vi "Rotation stage shgv2.vi"() -> ()   [LabVIEW 2020]
doc: "Shows how to move a motor to an absolute position."
uses:
  <vilib>/Utility/error.llb/DialogType.ctl
  <vilib>/DAQmx/read.llb/DAQmx Read (Counter 1D U32 1Chan NSamp).vi
  <vilib>/DAQmx/create/channels.llb/DAQmx Create Channel (CI-Period).vi
  <vilib>/DAQmx/create/channels.llb/DAQmx Create Channel (CO-Pulse Generation-Frequency).vi
  <vilib>/DAQmx/configure/timing.llb/DAQmx Timing (Implicit).vi
  <vilib>/DAQmx/miscellaneous.llb/DAQmx Fill In Error Info.vi
  <resource>/objmgr/daqmx.rc
panel:
  in  "Duty Cycle":dbl=0.5 format="%.6f"
  out "Input.BufSize":u32=1000000 format="%.0p"
  out "data":u32[](graph)
  out "Consumer Iteration 2":i32=1109257
  in  "stop 3":bool
  in  "number of samples per channel 2":i32=5000
  out "Producer Iteration 2":i32=1109256
  out "error out 2":errorcluster
  out "Loop Time (ms) 2":u32=10
  in  "dwell time (ms)":dbl=1.0 format="%.6f"
  in  "Photon Input (PFI)":tag="/Dev1/PFI0"
  in  "Rotation Angle (Degrees)":dbl=100.0 min=0.0
  in  "MG17Motor":refnum<k7>(container)
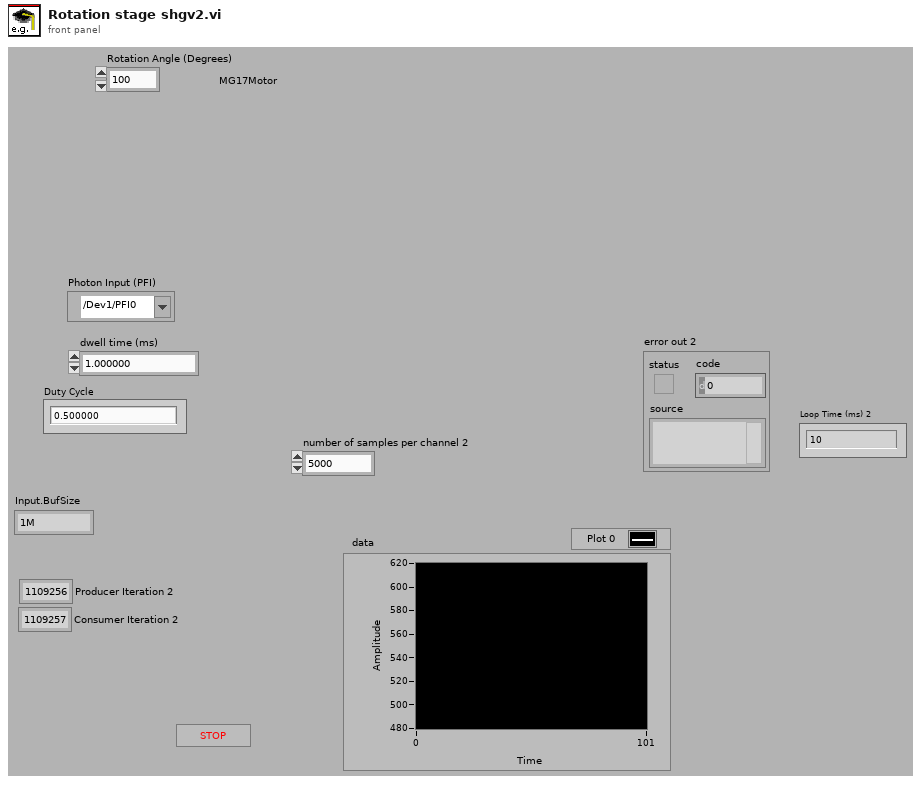
[diagram p1: front panel]
types:
  T1 = enum16{"open", "open or create", "create or replace", "create", "open (read-only)"}
  T2 = typedef "DialogType.ctl" = u16
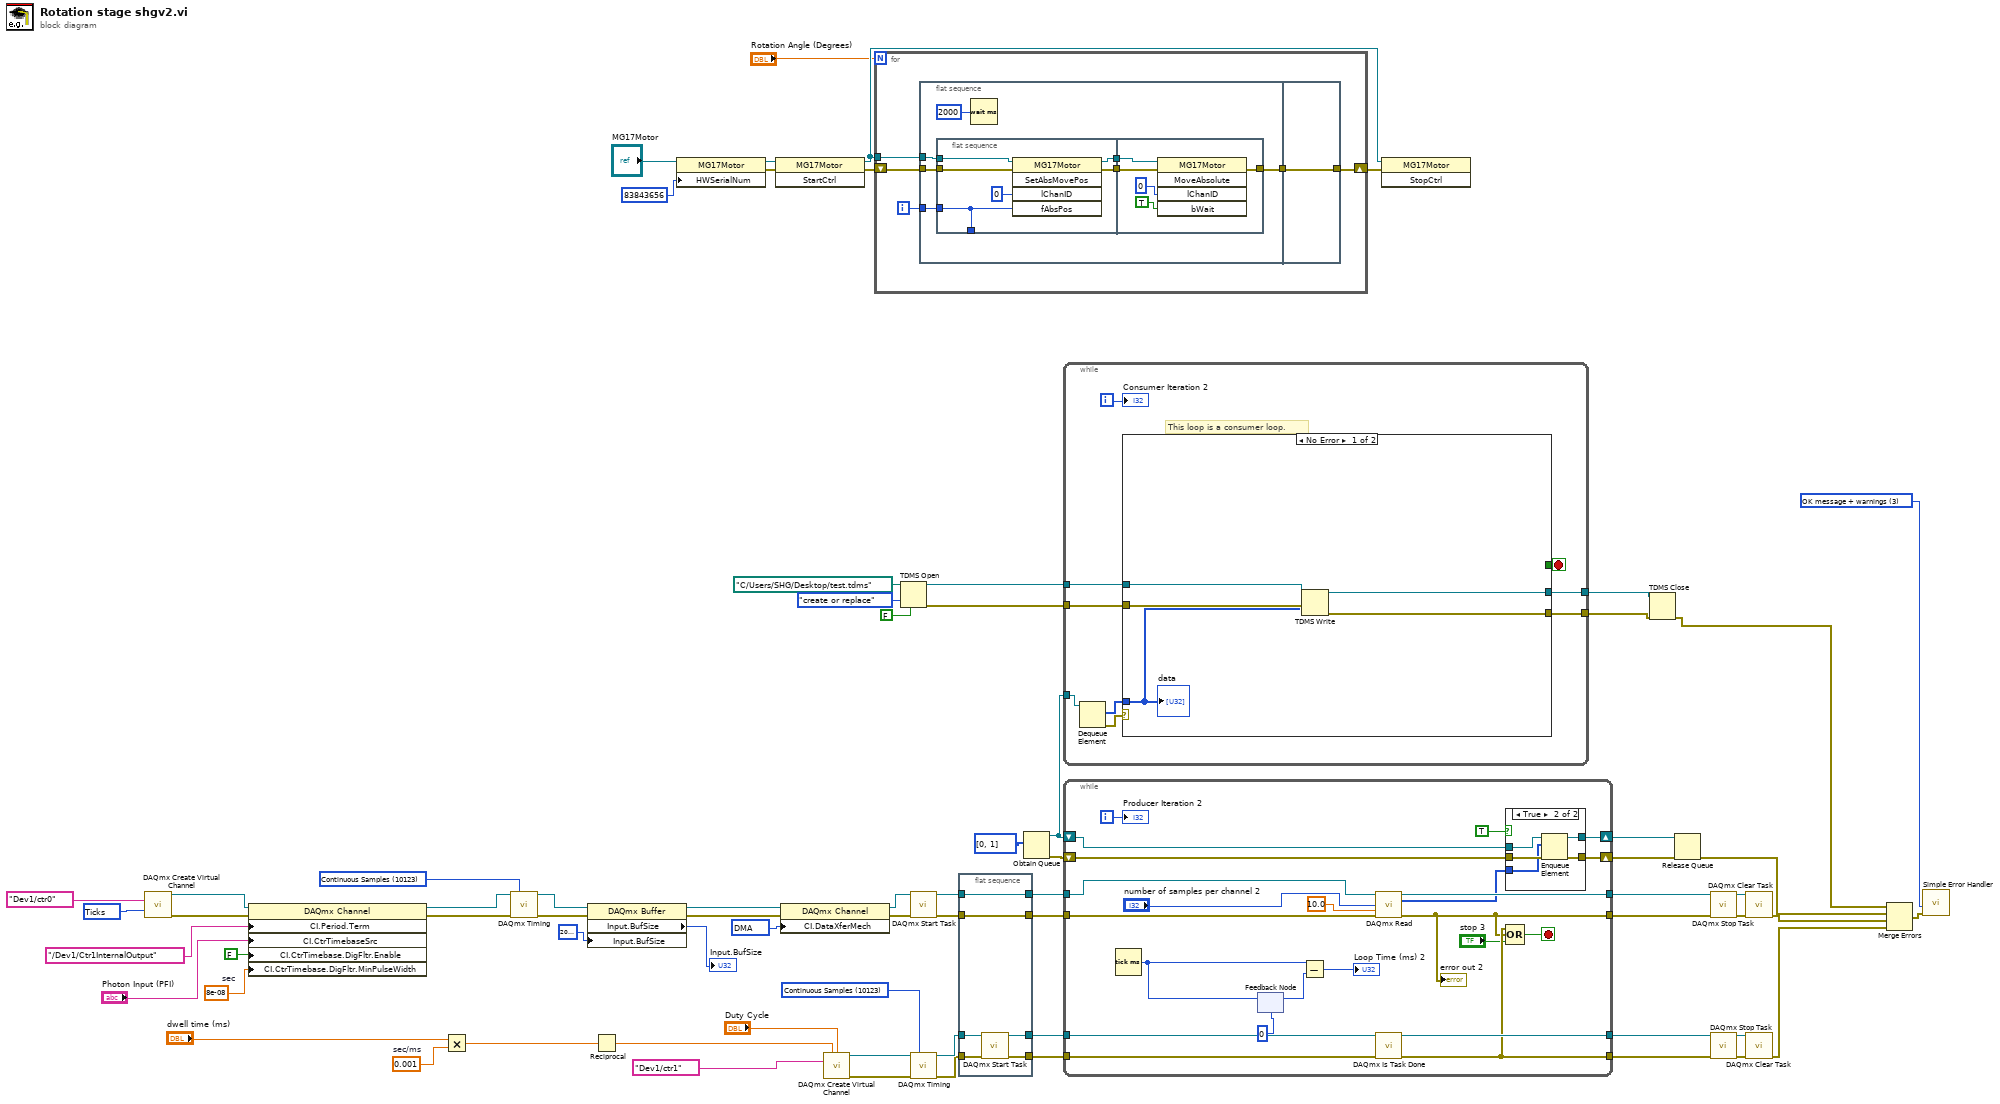
[diagram p0: block diagram]
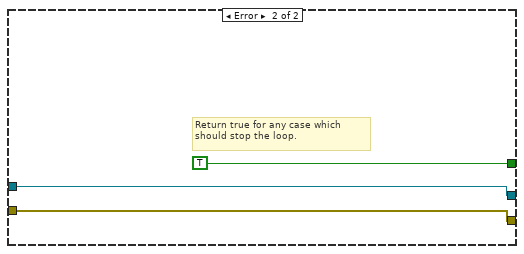
[diagram p2: hidden frame]
diagram:
  w9 = T2 3 items=["no dialog", "OK message", "continue or stop message", "OK message + warnings", "continue/stop + warnings"] ("type of dialog (OK msg:1)")
  w14 = 8e-08  # sec
  w25 = 10054 items=["DMA"=10054, "Interrupts"=10204, "Programmed I/O"=10264, "USB Bulk"=12590] ("CI.DataXferMech")
  w45 = 0.001  # sec/ms
  w55 = 10304 items=["Seconds"=10364, "Ticks"=10304, "From Custom Scale"=10065] ("units")
  w56 = 10123 items=["Finite Samples"=10178, "Continuous Samples"=10123, "Hardware Timed Single Point"=12522] ("sample mode")
  w57 = 10123 items=["Finite Samples"=10178, "Continuous Samples"=10123, "Hardware Timed Single Point"=12522] ("sample mode")
  n1 = call-poly <vilib>:"DAQmx Create Virtual Channel.vi"("counter"=tag "Dev1/ctr0", "units"=w55) -> ("task out"=w52:refnum<k21>, "error out"=w51:errorcluster)  [unwired: 12 in]
  n2 = property class="DAQmx Channel"(reference=w52, error in=w51, "CI.Period.Term"=tag "/Dev1/Ctr1InternalOutput", "CI.CtrTimebaseSrc"="Photon Input (PFI)", "CI.CtrTimebase.DigFltr.Enable"=FALSE, "CI.CtrTimebase.DigFltr.MinPulseWidth"=w14) -> (reference out=w50:refnum<k21>, error out=w49:errorcluster)
  n3 = Multiply(x="dwell time (ms)", y=w45) -> (x*y=w44:dbl)
  n4 = call-poly <vilib>:"DAQmx Timing.vi"("task/channels in"=w50, "sample mode"=w56, "error in"=w49) -> ("task out"=w20:refnum<k21>, "error out"=w19:errorcluster)  [unwired: 11 in]
  n5 = property class="DAQmx Buffer"(reference=w20, error in=w19, "Input.BufSize"=u32 2000000 ("samples per channel")) -> (reference out=w24:refnum<k21>, error out=w22:errorcluster, "Input.BufSize"=→"Input.BufSize":u32)
  n6 = Reciprocal(x=w44) -> (1/x=w43:dbl)
  n7 = property class="MG17Motor"(reference="MG17Motor", "HWSerialNum"=83843656) -> (reference out=w67:refnum<k7>, error out=w66:errorcluster)  [unwired: 1 in]
  n8 = invoke class="MG17Motor" method="StartCtrl"(reference=w67, error in=w66) -> (reference out=w71:refnum<k7>, error out=w70:errorcluster)  [unwired: 1 in, 1 out]
  n9 = property class="DAQmx Channel"(reference=w24, error in=w22, "CI.DataXferMech"=w25) -> (reference out=w18:refnum<k21>, error out=w17:errorcluster)
  n10 = call-poly <vilib>:"DAQmx Create Virtual Channel.vi"("frequency"=w43, "duty cycle"="Duty Cycle", "counter"=tag "Dev1/ctr1") -> ("task out"=w62:refnum<k21>, "error out"=w63:errorcluster)  [unwired: 11 in]
  n11 = for {
    N: "Rotation Angle (Degrees)" -> [_]
    tunnel: w71 -> [w76]
    shift-right: [w74] -> w69
    shift-left: w70 -> [w75]
    i -> [w72]
    n12 = flat-sequence {
      tunnel: w76 -> [w81]
      tunnel: w75 -> [w79]
      tunnel: [w78] -> w73
      tunnel: w72 -> [w80]
      tunnel: [w95] -> w74
      tunnel: w73 -> [w95]
      frame #0 {
        n13 = flat-sequence {
          tunnel: [w84] -> _
          tunnel: w79 -> [w88]
          tunnel: w81 -> [w87]
          tunnel: [w86] -> w83
          tunnel: [w85] -> w82
          tunnel: w80 -> [w84]
          tunnel: w83 -> [w92]
          tunnel: w82 -> [w91]
          tunnel: [w90] -> w78
          frame #0 {
            n14 = invoke class="MG17Motor" method="SetAbsMovePos"(reference=w87, error in=w88, "lChanID"=0, "fAbsPos"=w84) -> (reference out=w85:refnum<k7>, error out=w86:errorcluster)  [unwired: 1 in, 3 out]
          }
          frame #1 {
            n15 = invoke class="MG17Motor" method="MoveAbsolute"(reference=w91, error in=w92, "lChanID"=0, "bWait"=TRUE) -> (error out=w90:errorcluster)  [unwired: 1 in, 4 out]
          }
        }
        n16 = Wait (ms)(milliseconds to wait=u32 2000) -> ()  [unwired: 1 out]
      }
      frame #1 {
      }
    }
  }
  n17 = TDMS Open(6:FALSE ("disable buffering? (T)"), 10:T1."create or replace" ("operation (0:open)"), 11:path "C:/Users/SHG/Desktop/test.tdms" ("file path")) -> (0:w11:errorcluster, 3:w13:refnum<k34>)  [unwired: 4 in]
  n18 = call <vilib>:"DAQmx Start Task.vi"("task/channels in"=w18, "error in"=w17) -> ("task out"=w42:refnum<k21>, "error out"=w41:errorcluster)  [unwired: 12 in]
  n19 = call-poly <vilib>:"DAQmx Timing.vi"("task/channels in"=w62, "sample mode"=w57, "error in"=w63) -> ("task out"=w61:refnum<k21>, "error out"=w60:errorcluster)  [unwired: 11 in]
  n20 = flat-sequence {
    tunnel: w61 -> [w101]
    tunnel: w60 -> [w100]
    tunnel: [w99] -> w28
    tunnel: [w98] -> w29
    tunnel: w42 -> [w96]
    tunnel: w41 -> [w97]
    tunnel: [w97] -> w31
    tunnel: [w96] -> w30
    frame #0 {
      n21 = call <vilib>:"DAQmx Start Task.vi"("task/channels in"=w101, "error in"=w100) -> ("task out"=w98:refnum<k21>, "error out"=w99:errorcluster)  [unwired: 12 in]
    }
  }
  n22 = Obtain Queue(element data type=u32[] [0, 1] ("data")) -> (queue out=w40:refnum<queue>, error out=w39:errorcluster)  [unwired: 4 in, 1 out]
  n23 = while {
    tunnel: w40 -> [w110]
    tunnel: w13 -> [w105]
    tunnel: [w104] -> w12
    tunnel: w11 -> [w103]
    tunnel: [w102] -> w10
    i -> [w106]
    stop <- w107 stop-if-true
    # "This loop is a consumer loop."
    n24 = Dequeue Element(queue=w110) -> (element=w108:u32[], error out=w109:errorcluster)  [unwired: 2 in, 2 out]
    n25 = case shown="No Error" w109 {
      tunnel: w108 -> [w111 _]
      tunnel: [_ TRUE] -> w107
      tunnel: w105 -> [w115 w117]
      tunnel: [w114 w117] -> w104
      tunnel: w103 -> [w113 w116]
      tunnel: [w112 w116] -> w102
      frame No Error {
        n26 = TDMS Write(0:w115, 9:w111, 11:w113) -> (4:w114:refnum<k34>, 15:w112:errorcluster)  [unwired: 3 in, 2 out]
        "data" <- w111
      }
      frame Error {
        # "Return true for any case which should stop the loop."
      }
    }
    "Consumer Iteration 2" <- w106
  }
  n27 = while {
    shift-right: [w130] -> w37
    shift-left: w39 -> [w139]
    shift-right: [w140] -> w38
    shift-left: w40 -> [w141]
    tunnel: [w137] -> w34
    tunnel: [w125] -> w33
    tunnel: w31 -> [w136]
    tunnel: w30 -> [w135]
    tunnel: w29 -> [w129]
    tunnel: w28 -> [w128]
    tunnel: [w127] -> w27
    tunnel: [w126] -> w26
    i -> [w131]
    stop <- w123 stop-if-true
    n28 = Tick Count (ms)() -> (millisecond timer value=w122:u32)
    n29 = feedback #1(u32 0 ("millisecond timer value")) -> (w121:u32)
    n30 = feedback-in #1(w122) -> ()
    n31 = Subtract(x=w122, y=w121) -> (x-y=→"Loop Time (ms) 2":u32)
    n32 = call-poly <vilib>:"DAQmx Read.vi"("task/channels in"=w135, "number of samples per channel"="number of samples per channel 2", "timeout"=10.0, "error in"=w136) -> ("task out"=w137:refnum<k21>, "data"=w134:u32[], "error out"=w125:errorcluster)  [unwired: 9 in]
    "error out 2" <- w125
    n33 = call <vilib>:"DAQmx Is Task Done.vi"("task/channels in"=w129, "error in"=w128) -> ("task out"=w127:refnum<k21>, "error out"=w126:errorcluster)  [unwired: 11 in, 1 out]
    n34 = case shown="True" TRUE ("Case Constant\n(See Context Help)") {
      tunnel: w141 -> [w143 w148]
      tunnel: [w143 w147] -> w140
      tunnel: w139 -> [w142 w146]
      tunnel: [w142 w145] -> w130
      tunnel: w134 -> [_ w144]
      frame False {
      }
      frame True {
        n35 = Enqueue Element(queue=w148, element=w144, error in (no error)=w146) -> (queue out=w147:refnum<queue>, error out=w145:errorcluster)  [unwired: 1 in, 1 out]
      }
    }
    n36 = Compound Arithmetic op=OR(w126, w125, "stop 3") -> (w123:bool)
    "Producer Iteration 2" <- w131
  }
  n37 = invoke class="MG17Motor" method="StopCtrl"(reference=w71, error in=w69) -> ()  [unwired: 1 in, 3 out]
  n38 = TDMS Close(8:w10, 11:w12) -> (0:w5:errorcluster)  [unwired: 1 out]
  n39 = Release Queue(queue=w38, error in (no error)=w37) -> (error out=w4:errorcluster)  [unwired: 1 in, 2 out]
  n40 = call <vilib>:"DAQmx Stop Task.vi"("task/channels in"=w34, "error in"=w33) -> ("task out"=w35:refnum<k21>, "error out"=w36:errorcluster)  [unwired: 12 in]
  n41 = call <vilib>:"DAQmx Stop Task.vi"("task/channels in"=w27, "error in"=w26) -> ("task out"=w59:refnum<k21>, "error out"=w58:errorcluster)  [unwired: 12 in]
  n42 = call <vilib>:"DAQmx Clear Task.vi"("task in"=w35, "error in"=w36) -> ("error out"=w3:errorcluster)  [unwired: 13 in]
  n43 = call <vilib>:"DAQmx Clear Task.vi"("task in"=w59, "error in"=w58) -> ("error out"=w2:errorcluster)  [unwired: 13 in]
  n44 = Merge Errors(w5, w4, w3, w2) -> (w8:errorcluster)
  n45 = call <vilib>:"Simple Error Handler.vi"("type of dialog (OK msg:1)"=w9, "error in (no error)"=w8) -> ()  [unwired: 3 in, 5 out]
